vi "Moderate Turret Microswitches.vi"(1 "TurretRightMS":bool, 2 "Input":dbl, 3 "TurretLeftMS":bool) -> (0 "Output":dbl)   [LabVIEW 2011]
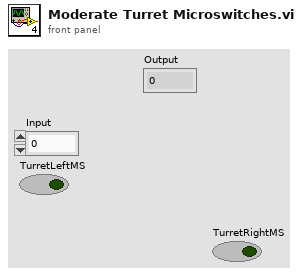
[diagram p1: front panel]
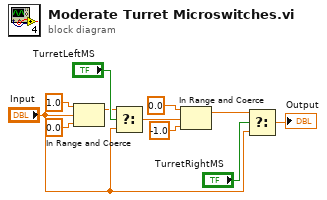
[diagram p0: block diagram]
diagram:
  n1 = In Range and Coerce(upper limit=1.0, x="Input", lower limit=0.0 ("x")) -> (coerced(x)=w8:dbl)  [unwired: 1 out]
  n2 = Select(t=w8, s="TurretLeftMS", f="Input") -> (s? t:f=w3:dbl)
  n3 = In Range and Coerce(upper limit=0.0, x=w3, lower limit=-1.0 ("x")) -> (coerced(x)=w7:dbl)  [unwired: 1 out]
  n4 = Select(t=w7, s="TurretRightMS", f="Input") -> (s? t:f=→"Output":dbl)
